vi "Error Handler.vi"(8 "error in (no error)":errorcluster, 10 "stop":bool, 11 "Plugin Thread in":refnum<class "Plugin Thread.lvclass">) -> (0 "error out":errorcluster, 2 "stop":bool, 3 "Plugin Thread out":refnum<class "Plugin Thread.lvclass">)   [LabVIEW 2017, in "DSF Core.lvlib" / "Plugin Thread.lvclass"]
uses:
  Thread/Plugin/Plugin Thread.lvclass
  C:/Users/Admin/Desktop/Data Sharing Framework/Source/Core/Engine/Classes/Thread/Thread.lvclass
  Thread/Plugin/Plugin Thread.lvclass/Plugin Thread.ctl
  Interfaces/Transceiver Interface/Write Plugin Error.vi
  Interfaces/Transceiver Interface/Plugin Interface.lvclass
  Thread/Thread.lvclass
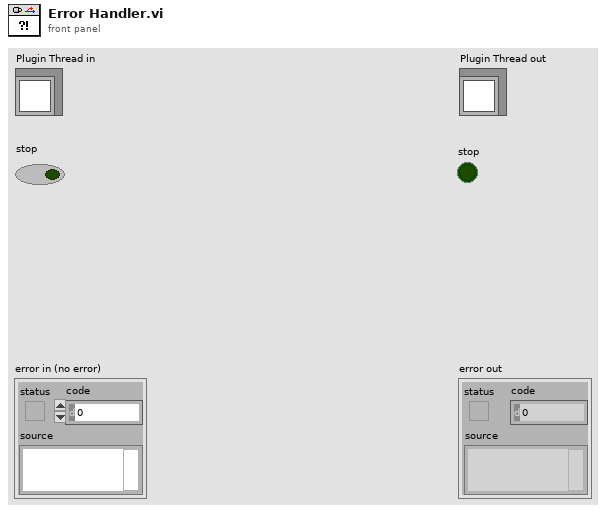
[diagram p1: front panel]
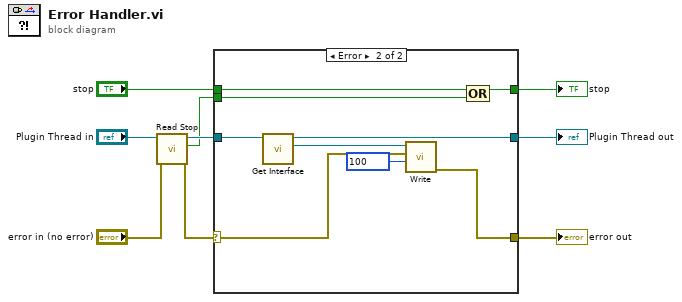
[diagram p0: block diagram]
diagram:
  n1 = call "Read Stop.vi"("error in (no error)"="error in (no error)", "Thread in"="Plugin Thread in") -> ("error out"=w2:errorcluster, "stop"=w1:bool, "Thread out"=w4:refnum<class "Plugin Thread.lvclass">)  [unwired: 7 in]
  n2 = case shown="Error" w2 {
    selector: w2 -> [w12 w15]
    tunnel: "stop" -> [w11 w17]
    tunnel: [w12 w13] -> w8
    tunnel: [w11 w16] -> w7
    tunnel: w4 -> [w10 w21]
    tunnel: [w10 w20] -> w6
    tunnel: w1 -> [_ w14]
    frame No Error {
    }
    frame Error {
      n3 = call "Get Interface.vi"("Transceiver Thread in"=w21) -> ("Interface"=w19:refnum<class "Plugin Interface.lvclass">, "Transceiver Thread out"=w20:refnum<class "Plugin Thread.lvclass">)  [unwired: 9 in]
      n4 = call-poly "Write.vi"("timeout in ms (0)"=100, "error"=w15, "Plugin Interface in"=w19) -> ("error out"=w13:errorcluster)  [unwired: 7 in, 1 out]
      n5 = Compound Arithmetic op=OR(w17, w14) -> (w16:bool)
    }
  }
  "error out" <- w8
  "Plugin Thread out" <- w6
  "stop" <- w7
